vi "Control to Sample Container.vi"(8 "error in (no error)":errorcluster, 11 "Sample Container Ref":refnum<vi>) -> (0 "error out":errorcluster, 3 "Sample Container":T1)   [LabVIEW 2015]
uses:
  Controls/Sample Container.ctl
  Sample/Sample.lvclass
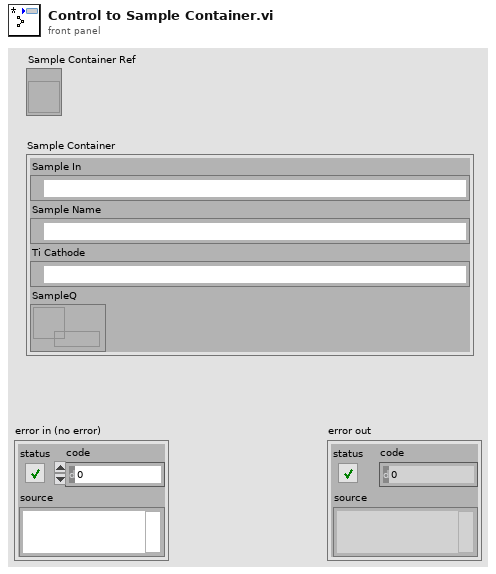
[diagram p1: front panel]
types:
  T1 = typedef "Sample Container.ctl" = cluster{"Sample In":refnum<k21>, "Sample Name":refnum<k21>, "Ti Cathode":refnum<k21>, "SampleQ":refnum<queue>}
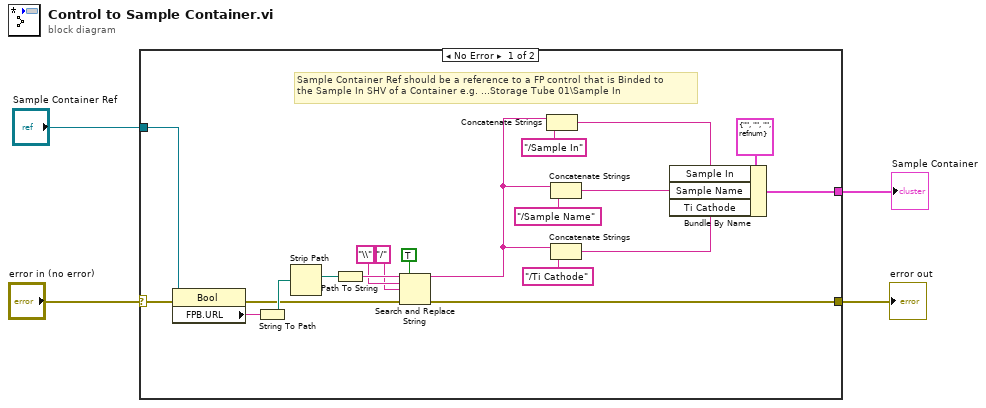
[diagram p0: block diagram]
diagram:
  n1 = case shown="No Error" "error in (no error)" {
    selector: "error in (no error)" -> [w24 w25]
    tunnel: [w10 w25] -> w3
    tunnel: "Sample Container Ref" -> [w23 _]
    tunnel: [w11 _] -> w2
    frame No Error {
      # "Sample Container Ref should be a reference to a FP control that is Binded to\nthe Sample In SHV of a Container e.g. ...Storage Tube 01\\Sample In"
      n2 = property class="Bool"(reference=w23, error in=w24) -> (error out=w14:errorcluster, "FPB.URL"=w22:string)  [unwired: 1 out]
      n3 = String To Path(string=w22) -> (path=w21:path)
      n4 = Strip Path(path=w21) -> (stripped path=w20:path)  [unwired: 1 out]
      n5 = Path To String(path=w20) -> (string=w19:string)
      n6 = Search and Replace String(replace all?=TRUE ("replace all? (F)"), input string=w19, search string="\\", replace string="/" ("replace string (\"\")"), error in=w14) -> (result string=w8:string, error out=w10:errorcluster)  [unwired: 3 in, 2 out]
      n7 = Concatenate Strings(w8, "/Sample In" ("string")) -> (w5:string)
      n8 = Concatenate Strings(w8, "/Sample Name" ("name or relative path")) -> (w6:string)
      n9 = Concatenate Strings(w8, "/Ti Cathode" ("name or relative path")) -> (w15:string)
      n10 = Bundle By Name(cluster=T1 {"Sample In"="", "Sample Name"="", "Ti Cathode"="", "SampleQ"=refnum} ("Sample Container"), "Sample In"=w5, "Sample Name"=w6, "Ti Cathode"=w15) -> (w11:T1)
    }
    frame Error {
    }
  }
  "error out" <- w3
  "Sample Container" <- w2
